vi "Categorize Terminals and Names.vi"(10 "terminal names":string[](array[string]), 11 "terminal addresses":T1[](array[typedef])) -> (1 "map from terminal address (string) to terminal name":map{string, string}(c390), 2 "remote terminals":string[](array[string]), 3 "bus controller":string[](array[string]))   [LabVIEW 2020, in "Ballard MIL-STD-1553 System Explorer.lvlib" / "Implementation.lvlib" / "Refresh.lvlib"]
uses:
  Refresh.lvlib
  Shared/Address.ctl
  Scripting/Ballard MIL-STD-1553 Scripting.lvlib
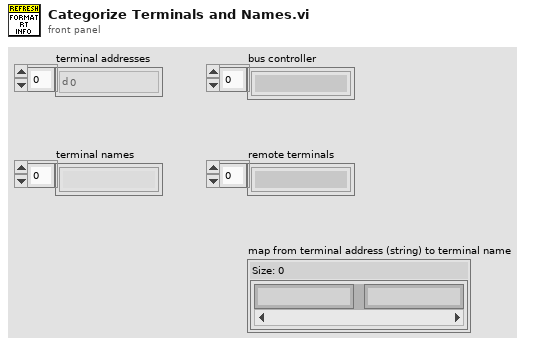
[diagram p1: front panel]
types:
  T1 = typedef "Address.ctl" = u16
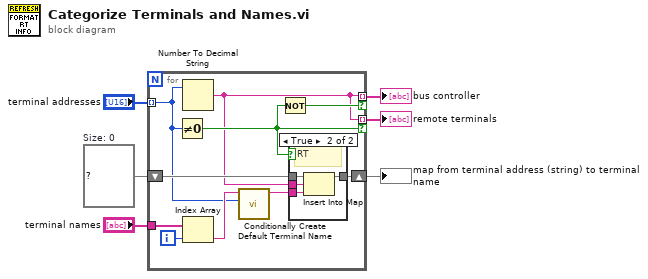
[diagram p0: block diagram]
diagram:
  w5 = map{string, string} {}  # Size: 0
  n1 = for {
    tunnel: "terminal addresses" -> [w7] mode=indexing
    tunnel: [w10] -> w1 mode=indexing if=w14
    tunnel: [w10] -> w4 mode=indexing if=w13
    tunnel: "terminal names" -> [w16]
    shift-right: [w11] -> w6
    shift-left: w5 -> [w12]
    i -> [w15]
    n2 = Not Equal To 0?(x=w7) -> (x != 0?=w13:bool)
    n3 = Number To Decimal String(number=w7) -> (decimal integer string=w10:string)  [unwired: 1 in]
    n4 = Index Array(array=w16, index=w15) -> (element=w9:string)
    n5 = call "Conditionally Create Default Terminal Name.vi"("terminal address in"=w7, "terminal name in"=w9) -> ("terminal name out"=w8:string)  [unwired: 8 in, 1 out]
    n6 = Not(x=w13) -> (.not. x?=w14:bool)
    n7 = case shown="True" w13 {
      tunnel: w8 -> [_ w20]
      tunnel: w12 -> [w17 w21]
      tunnel: [w17 w18] -> w11
      tunnel: w10 -> [_ w19]
      frame False {
        # "BC"
      }
      frame True {
        # "RT"
        n8 = Insert Into Map(map in=w21, key=w19, value=w20) -> (map out=w18:map{string, string})  [unwired: 2 out]
      }
    }
  }
  "map from terminal address (string) to terminal name" <- w6
  "remote terminals" <- w4
  "bus controller" <- w1
